vi "TCPClient1.vi"() -> ()   [LabVIEW 2013]
uses:
  <vilib>/Utility/error.llb/DialogType.ctl
panel:
  out "bytes written":i32
  in  "data in":string
  out "data out 2":string
  in  "Disconnect":bool caption="Disconn"
  out "Connected":bool
  out "message":string=" INSTRUCTIONS:\r\rNormal Use:  When using subVIs that incorporate the error in/error out (or error I/O) structure, place this handler where you want to inform the user of an error, typically at the end of the I/O data path, as the last action of the program.  If the error in error? is ERROR, the handler creates a message describing the error and its source.  If the type of dialog = 1 (default), the message is displayed to the user, who can only acknowedge it.  If the type = 2, the user can acknowledge the message or abort execution; aborting a program with active I/O is not recommended.  If the type = 0, no message is displayed; this is used to process the error programmatically, and the error out cluster elements are wired to individual terminals for that reason.  \r\rOther Use:\n\r\nlocal testing.  To test the error code of a subVI or function that does not have the error I/O structure, you can wire its error code and a source string to the local error code and error source inputs.  If error in error? indicates no error and error code is not equal to 0, the local code and source are substituted for the error in values, and error? is set TRUE (ERROR)."
  in  "Connect":bool
  out "I":i32
  in  "bytes to read":i32
  out "data out":string
  in  "stop":bool
  in  "порт":u16=4001
  in  "IP-адрес":string="192.168.127.254"
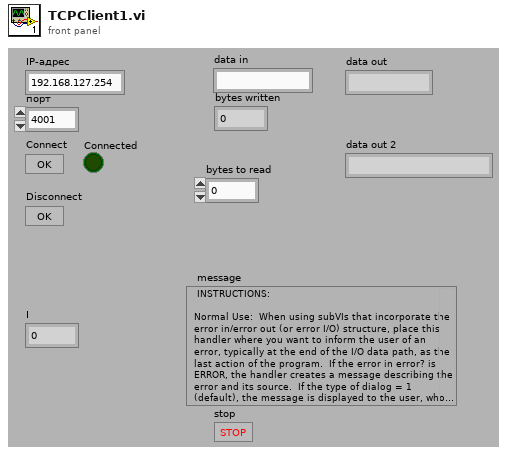
[diagram p1: front panel]
types:
  T1 = enum16{"Standard", "Buffered", "CRLF", "Immediate"}
  T2 = typedef "DialogType.ctl" = u16
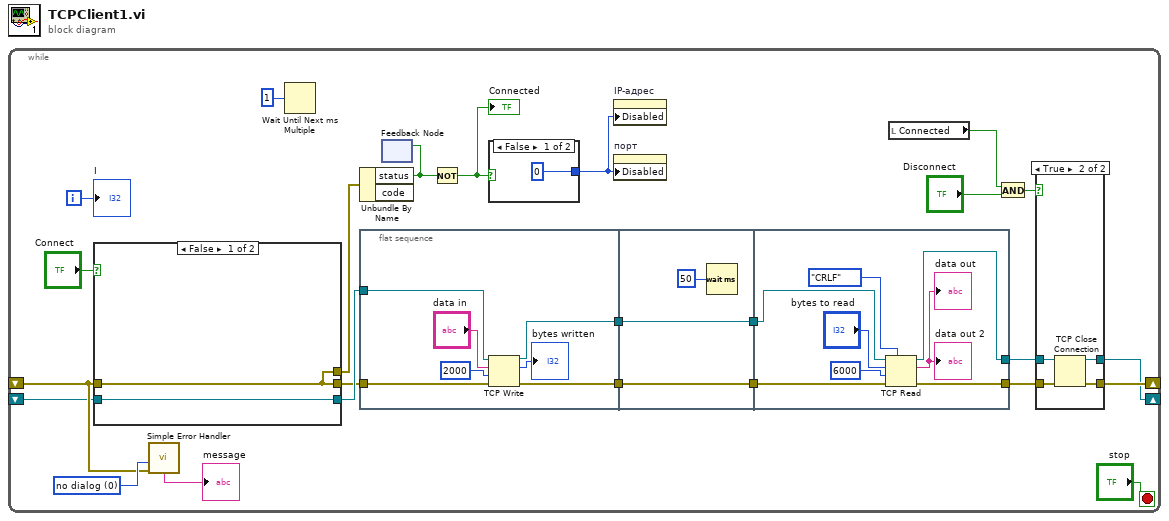
[diagram p0: block diagram]
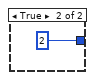
[diagram p2: hidden frame]
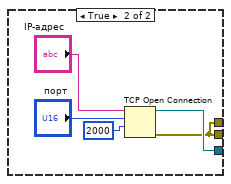
[diagram p4: hidden frame]
diagram:
  n1 = while {
    shift-right: [w6] -> _
    shift-left: _ -> [w7]
    shift-right: [w4] -> _
    shift-left: _ -> [w5]
    i -> [w18]
    stop <- "stop" stop-if-true
    w15 = T2 0 items=["no dialog", "OK message", "continue or stop message", "OK message + warnings", "continue/stop + warnings"] ("type of dialog (OK msg:1)")
    n2 = case shown="False" "Connect" {
      tunnel: [w35 w38] -> w22
      tunnel: [w34 w37] -> w21
      tunnel: w5 -> [w35 _]
      tunnel: w7 -> [w34 _]
      tunnel: [w34 w37] -> w19
      frame False {
      }
      frame True {
        n3 = TCP Open Connection(address="IP-адрес", remote port or service name="порт", timeout ms (60000)=u32 2000 ("millisecond multiple")) -> (connection ID=w38:refnum<k5>, error out=w37:errorcluster)  [unwired: 1 in, 1 out]
      }
    }
    n4 = call <vilib>:"Simple Error Handler.vi"("type of dialog (OK msg:1)"=w15, "error in (no error)"=w7) -> ("message"=→"message":string)  [unwired: 7 out]
    n5 = Wait Until Next ms Multiple(millisecond multiple=u32 1) -> ()  [unwired: 1 out]
    n6 = Unbundle By Name(w19) -> ("status"=w17:bool)  [unwired: 1 out]
    n7 = flat-sequence {
      tunnel: w22 -> [w47]
      tunnel: w21 -> [w46]
      tunnel: [w45] -> w3
      tunnel: [w44] -> w2
      tunnel: [w49] -> w24
      tunnel: [w50] -> w23
      tunnel: w3 -> [w50]
      tunnel: w2 -> [w49]
      tunnel: [w54] -> w13
      tunnel: [w53] -> w12
      tunnel: w24 -> [w56]
      tunnel: w23 -> [w55]
      frame #0 {
        n8 = TCP Write(connection ID=w47, data in="data in", error in (no error)=w46, 9:2000 ("timeout ms (25000)")) -> (connection ID out=w44:refnum<k5>, bytes written=→"bytes written":i32, error out=w45:errorcluster)
      }
      frame #1 {
        n9 = Wait (ms)(milliseconds to wait=u32 50) -> ()  [unwired: 1 out]
      }
      frame #2 {
        n10 = TCP Read(connection ID=w56, bytes to read="bytes to read", error in (no error)=w55, 7:T1."CRLF" ("mode (standard)"), 9:6000 ("timeout ms (25000)")) -> (connection ID out=w53:refnum<k5>, data out=→"data out" →"data out 2":string, error out=w54:errorcluster)
      }
    }
    n11 = feedback-in #1(w17) -> ()
    n12 = feedback #1() -> ()  [unwired: 2 out]
    n13 = Not(x=w17) -> (.not. x?=w9:bool)
    "Connected" <- w9
    n14 = case shown="False" w9 {
      tunnel: [u8 0 ("Disabled") u8 2 ("Disabled")] -> w8
      frame False {
      }
      frame True {
      }
    }
    n15 = property on="IP-адрес" class="Str"("Disabled"=w8) -> ()  [unwired: 2 in, 2 out]
    n16 = property on="порт" class="DigNum (strict)"("Disabled"=w8) -> ()  [unwired: 2 in, 2 out]
    n17 = local read "Connected"() -> (w10:bool)
    n18 = And(x=w10, y="Disconnect") -> (x .and. y?=w11:bool)
    n19 = case shown="True" w11 {
      tunnel: w13 -> [w29 w33]
      tunnel: [w29 w32] -> w6
      tunnel: w12 -> [w28 w31]
      tunnel: [w28 w30] -> w4
      frame False {
      }
      frame True {
        n20 = TCP Close Connection(connection ID=w31, error in (no error)=w33) -> (connection ID out=w30:refnum<k5>, error out=w32:errorcluster)  [unwired: 1 out]
      }
    }
    "I" <- w18
  }
